vi "5492_PixyToRPM.vi"(10 "Height":dbl) -> (3 "RPM":dbl)   [LabVIEW 2016]
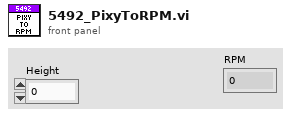
[diagram p1: front panel]
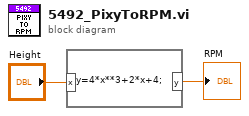
[diagram p0: block diagram]
diagram:
  n1 = formula code="y=4*x**3+2*x+4;"("x"="Height") -> ("y"=→"RPM":dbl)
